vi "Constructor.vi"(8 "error in (no error)":errorcluster, 11 "LatestValueCalculation in":refnum<class "LatestValueCalculation.lvclass">) -> (0 "error out":errorcluster, 3 "LatestValueCalculation out":refnum<class "LatestValueCalculation.lvclass">)   [LabVIEW 2015, in "LatestValueCalculation.lvclass"]
uses:
  Waveform-Processing-Custom-Device Configuration.llb/LatestValueCalculation.lvclass
  Waveform-Processing-Custom-Device Configuration.llb/WaveformCalculation.lvclass/WaveformCalculation.ctl
  Waveform-Processing-Custom-Device Configuration.llb/WaveformCalculation.lvclass
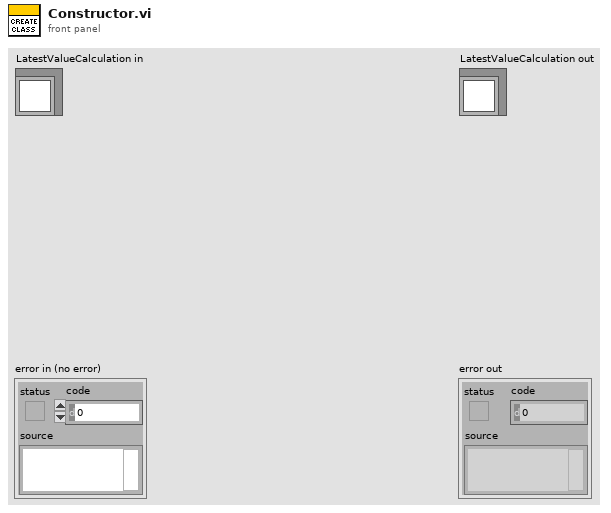
[diagram p1: front panel]
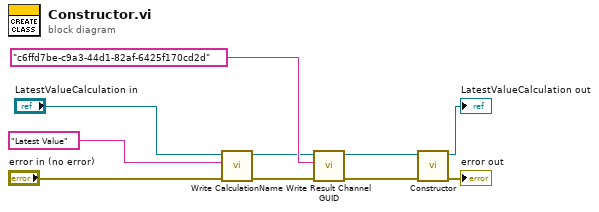
[diagram p0: block diagram]
diagram:
  n1 = call "Write CalculationName.vi"("error in (no error)"="error in (no error)", "CalculationName"="Latest Value", "WaveformCalculation in"="LatestValueCalculation in") -> ("error out"=w5:errorcluster, "WaveformCalculation out"=w2:refnum<class "LatestValueCalculation.lvclass">)  [unwired: 7 in]
  n2 = call "Write Result Channel GUID.vi"("error in (no error)"=w5, "Result Channel GUID"="c6ffd7be-c9a3-44d1-82af-6425f170cd2d", "WaveformCalculation in"=w2) -> ("error out"=w4:errorcluster, "WaveformCalculation out"=w1:refnum<class "LatestValueCalculation.lvclass">)  [unwired: 7 in]
  n3 = call-parent "Constructor.vi"("error in (no error)"=w4, "WaveformCalculation in"=w1) -> ("error out"=→"error out":errorcluster, "WaveformCalculation out"=→"LatestValueCalculation out":refnum<class "LatestValueCalculation.lvclass">)  [unwired: 8 in]
